vi "ldpctest.vi"() -> ()   [LabVIEW 2013]
uses:
  <vilib>/addons/Modulation/Digital/Channel Coding/MT LDPC Decoder (Serial Schedule).vi
  <vilib>/imath/engines/lvmath2/RunTimeEngine/ErrorHandling/NIMS_Finalize Error.vi
  <vilib>/imath/engines/lvmath2/RunTimeEngine/NodeEndStatement/NIMS_NodeEndStatement_Output.vi
  <instcachedir>/0/NIMS_NodeEndStatement_Output_53EC0D466D134D7ABD903AC30B43404B.lvgen/NIMS_NodeEndStatement_Output_53EC0D466D134D7ABD903AC30B43404B_011.vi
  <instcachedir>/0/NIMS_NodeEndStatement_Output_53EC0D466D134D7ABD903AC30B43404B.lvgen/NIMS_NodeEndStatement_Output_53EC0D466D134D7ABD903AC30B43404B_004.vi
  <vilib>/imath/engines/lvmath2/RunTimeEngine/BuiltInFunctions/randint/NIMS_randint(1,I32,RV).vi
  <vilib>/imath/engines/lvmath2/RunTimeEngine/ErrorHandling/NIMS_Create Error From Enums.vi
  <vilib>/imath/engines/lvmath2/RunTimeEngine/BuiltInFunctions/length/NIMS_length(GV).vi
  <instcachedir>/0/NIMS_length(GV)_08A3D13377FD4E4B96F5795FBF3698FA.lvgen/NIMS_length(GV)_08A3D13377FD4E4B96F5795FBF3698FA_002.vi
  <instcachedir>/0/NIMS_length(GV)_08A3D13377FD4E4B96F5795FBF3698FA.lvgen/NIMS_length(GV)_08A3D13377FD4E4B96F5795FBF3698FA_001.vi
  <vilib>/imath/engines/lvmath2/RunTimeEngine/BuiltInFunctions/zeros/NIMS_V=zeros(I32,I32).vi
  <vilib>/imathl/engines/lvmath/Functions/Error Handling/Create Error.vi
  <vilib>/imath/engines/lvmath2/RunTimeEngine/BuiltInFunctions/imag/NIMS_imag(Complex).vi
  <instcachedir>/0/NIMS_imag(Complex)_3180D40D00C843A49C2B33397F857BF3.lvgen/NIMS_imag(Complex)_3180D40D00C843A49C2B33397F857BF3_002.vi
  <instcachedir>/0/NIMS_NodeEndStatement_Output_53EC0D466D134D7ABD903AC30B43404B.lvgen/NIMS_NodeEndStatement_Output_53EC0D466D134D7ABD903AC30B43404B_005.vi
  <vilib>/imath/engines/lvmath2/RunTimeEngine/IndexReplace/NIMS V(R3)=V.vi
  <instcachedir>/0/NIMS V(R3)=V_69F337331DAD430986A98313EEA6EC3D.lvgen/NIMS V(R3)=V_69F337331DAD430986A98313EEA6EC3D_001.vi
  <vilib>/imath/engines/lvmath2/RunTimeEngine/BuiltInFunctions/abs/NIMS_abs(signed).vi
  <instcachedir>/0/NIMS_abs(signed)_C4FCB8E6058B49B797C7C8D53CA5F6EC.lvgen/NIMS_abs(signed)_C4FCB8E6058B49B797C7C8D53CA5F6EC_001.vi
  <instcachedir>/0/NIMS_NodeEndStatement_Output_53EC0D466D134D7ABD903AC30B43404B.lvgen/NIMS_NodeEndStatement_Output_53EC0D466D134D7ABD903AC30B43404B_018.vi
  <vilib>/addons/Modulation/niDMT.lvlib
panel:
  out "exp(x)":dbl[](array[numeric])
  out "LLR":dbl[](array[numeric])
  in  "n":i32=12
  out "size(s)":i32[](array[numeric])
  in  "j":i32=3
  in  "maximum number of iterations":i32=30
  out "number":i32
  in  "number of bits (per block)":dbl
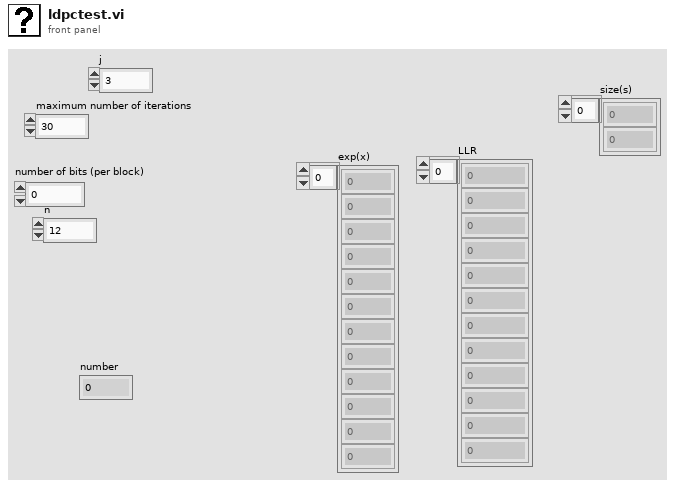
[diagram p1: front panel]
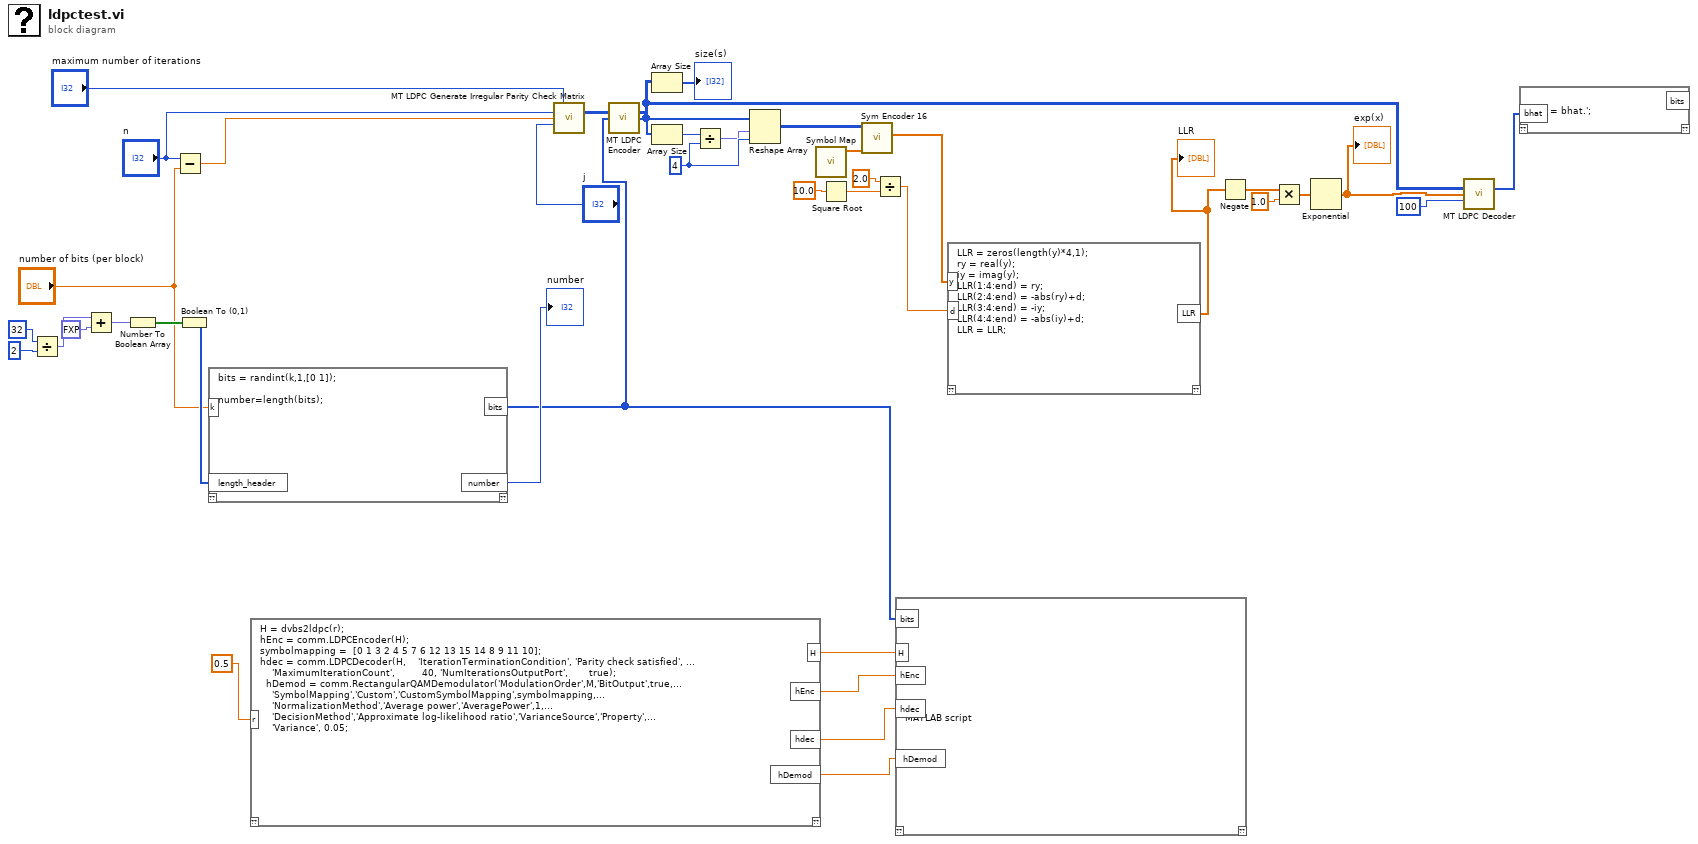
[diagram p0: block diagram]
diagram:
  w30 = 4 ("dimension size")
  n1 = Divide(x=32, y=2) -> (x/y=w38:fxp<+,9,9>)
  n2 = Add(x=w38, y=fxp<+,9,9> 5.0) -> (x+y=w35:fxp<+,10,10>)
  n3 = Number To Boolean Array(number=w35) -> (Boolean array=w40:bool[])
  n4 = Subtract(x="n", y="number of bits (per block)") -> (x-y=w34:dbl)
  n5 = Boolean To (0,1)(Boolean=w40) -> (0, 1=w12:i16[])
  n6 = mathscript code="bits = randint(k,1,[0 1]);\n\nnumber=length(bits);"("k"="number of bits (per block)", "length_header"=w12) -> ("bits"=w5:i32[], "number"=→"number":i32)  [unwired: 1 in, 1 out]
  n7 = script code="H = dvbs2ldpc(r);\nhEnc = comm.LDPCEncoder(H);\nsymbolmapping =  [0 1 3 2 4 5 7 6 12 13 15 14 8 9 11 10];\nhdec = comm.LDPCDecoder(H,    'IterationTerminationCondition', 'Parity check satisfied', ...\n    'MaximumIterationCount',         40, 'NumIterationsOutputPort',       true);\n  hDemod = comm.RectangularQAMDemodulator('ModulationOrder',M,'BitOutput',true,...\n    'SymbolMapping','Custom','CustomSymbolMapping',symbolmapping,...\n    'NormalizationMethod','Average power','AveragePower',1,... \n    'DecisionMethod','Approximate log-likelihood ratio','VarianceSource','Property',...\n    'Variance', 0.05;"("r"=0.5 ("Real")) -> ("H"=w4:dbl, "hEnc"=w3:dbl, "hdec"=w2:dbl, "hDemod"=w1:dbl)  [unwired: 1 in, 1 out]
  n8 = call <vilib>:"MT LDPC Generate Irregular Parity Check Matrix.vi"("maximum number of iterations"="maximum number of iterations", "n"="n", "m"=w34, "j"="j") -> ("irregular parity check matrix"=w32:i8[][])  [unwired: 10 in, 1 out]
  n9 = call <vilib>:"MT LDPC Encoder.vi"("parity check matrix in"=w32, "input bit stream"=w5) -> ("parity check matrix out"=w17:i8[][], "output bit stream"=w26:i8[])  [unwired: 11 in, 1 out]
  n10 = Array Size(array=w17) -> (size(s)=→"size(s)":i32[])
  n11 = Array Size(array=w26) -> (size(s)=w28:i32)
  n12 = Divide(x=w28, y=w30) -> (x/y=w29:fxp<+,27,27>)
  n13 = Reshape Array(w26, w29, w30) -> (w27:i8[][])
  n14 = call "Symbol Map.vi"() -> ("symbol_map"=w20:cdb[])  [unwired: 11 in]
  n15 = Square Root(x=10.0) -> (sqrt(x)=w23:dbl)
  n16 = call "Sym Encoder 16.vi"("symbol_map"=w20, "b"=w27) -> ("a"=w9:cdb[])  [unwired: 9 in]
  n17 = Divide(x=2.0, y=w23) -> (x/y=w8:dbl)
  n18 = script code="MATLAB script"("H"=w4, "hEnc"=w3, "hdec"=w2, "bits"=w5, "hDemod"=w1) -> ()  [unwired: 1 in, 1 out]
  n19 = mathscript code="LLR = zeros(length(y)*4,1);\nry = real(y);\niy = imag(y);\nLLR(1:4:end) = ry;\nLLR(2:4:end) = -abs(ry)+d;\nLLR(3:4:end) = -iy;\nLLR(4:4:end) = -abs(iy)+d;\nLLR = LLR;"("y"=w9, "d"=w8) -> ("LLR"=w10:dbl[])  [unwired: 1 in, 1 out]
  "LLR" <- w10
  n20 = Negate(x=w10) -> (-x=w15:dbl[])
  n21 = Multiply(x=w15, y=1.0) -> (x*y=w19:dbl[])
  n22 = Exponential(1:w19) -> (0:w7:dbl[])
  "exp(x)" <- w7
  n23 = call-poly <vilib>:"MT LDPC Decoder.vi"("parity check matrix"=w17, "likelihoods"=w7, "maximum number of iterations"=100) -> ("output bit stream"=w14:i8[])  [unwired: 11 in, 1 out]
  n24 = mathscript code="bits = bhat.';"("bhat"=w14) -> ()  [unwired: 1 in, 2 out]
